vi "_PC_NS_SubVI_Signal_I162DBL.vi"(8 "error in (no error)":errorcluster, 10 "Int signal in":waveform(i16)) -> (0 "error out":errorcluster, 2 "SGL sigal out":waveform(sgl))   [LabVIEW 2018]
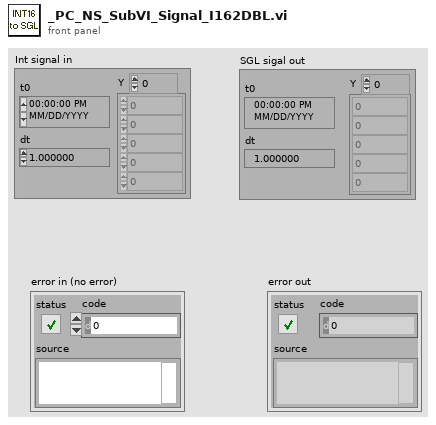
[diagram p1: front panel]
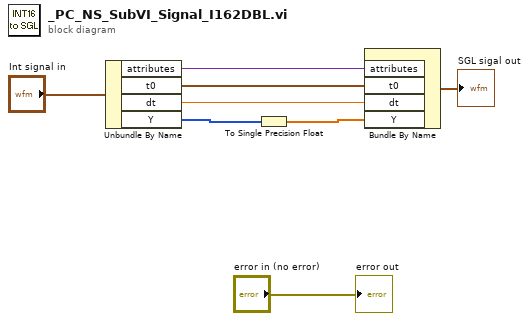
[diagram p0: block diagram]
diagram:
  n1 = Unbundle By Name("Int signal in") -> ("attributes"=w4:variant, "t0"=w5:timestamp, "dt"=w6:dbl, "Y"=w8:i16[])
  n2 = To Single Precision Float(number=w8) -> (single precision float=w2:sgl[])
  n3 = Bundle By Name("attributes"=w4, "t0"=w5, "dt"=w6, "Y"=w2) -> (→"SGL sigal out":waveform(sgl))  [unwired: 1 in]
  "error out" <- "error in (no error)"
